vi "4_oop.vi"() -> ()   [LabVIEW 2024]
uses:
  <vilib>/Python/Open Venv Python Session.vi
panel:
  in  "Place":string(combo)="Baden, CH"
  out "Temperature [°C]":dbl
  in  "stop":bool
  # "The Independent Graphical Developer Conference\n11-13 September 2024\nStuttgart, Germany"
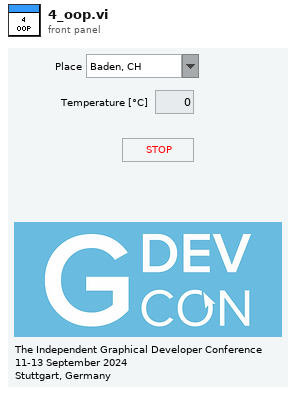
[diagram p1: front panel]
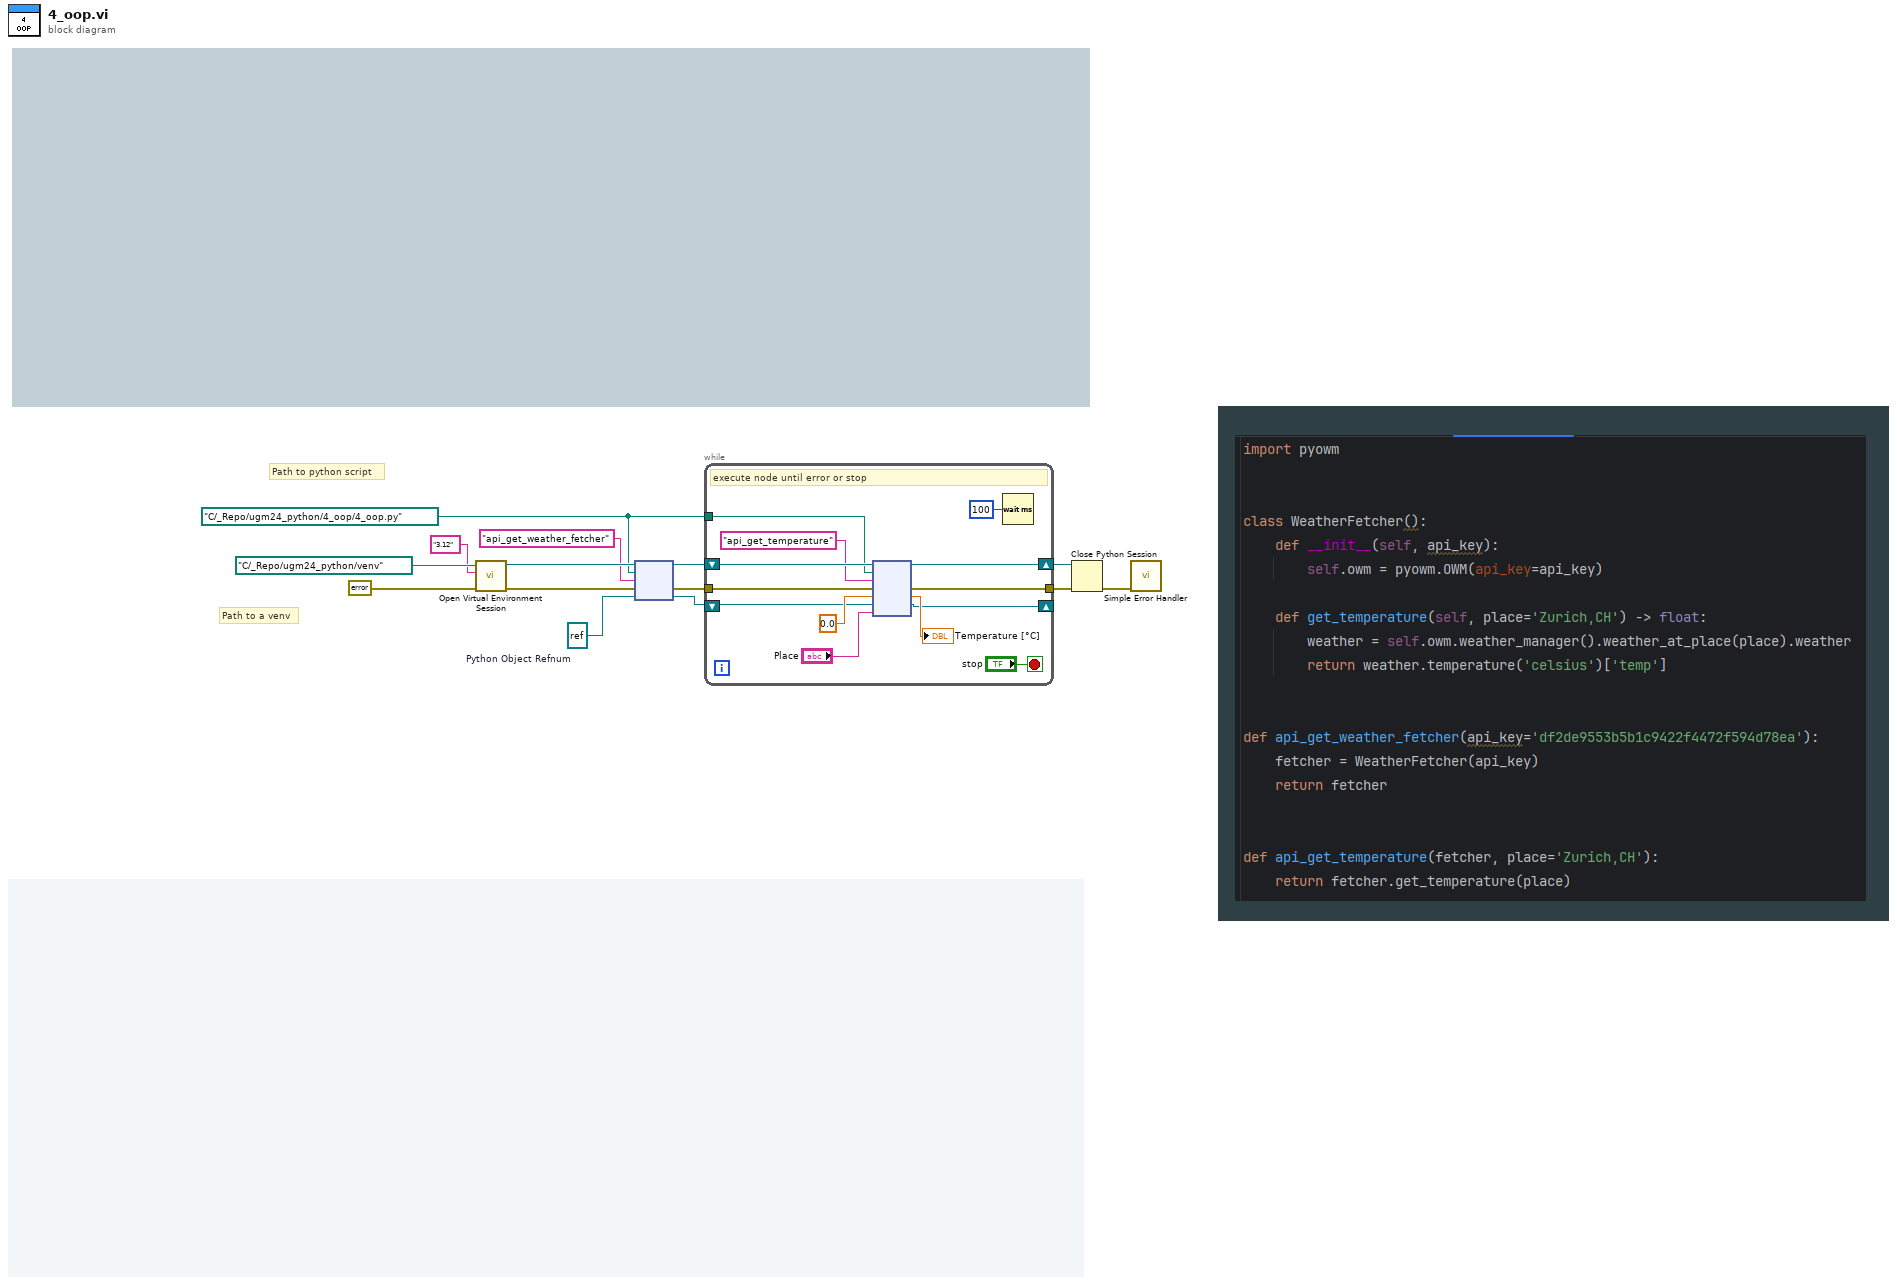
[diagram p0: block diagram]
diagram:
  w6 = refnum<k38> refnum  # Python Object Refnum
  w4 = path "C:/_Repo/ugm24_python/4_oop/4_oop.py" ("Path")
  # "Path to a venv"
  # "Path to python script"
  n1 = call-poly <vilib>:"Open Virtual Environment Session.vi"("error in (no error)"=errorcluster {"status"=FALSE, "code"=0, "source"=""}, "Python version"="3.12", "Env path"=path "C:/_Repo/ugm24_python/venv") -> ("error out"=w8:errorcluster, "session out"=w7:refnum<k35>)  [unwired: 7 in]
  n2 = node(w7, w4, "api_get_weather_fetcher" ("function name"), w8, w6) -> (w2:refnum<k35>, w3:errorcluster, w1:refnum<k38>)  [unwired: 2 out]
  n3 = while {
    tunnel: w3 -> [w27]
    tunnel: w4 -> [w25]
    tunnel: [w23] -> w14
    shift-right: [w22] -> w13
    shift-left: w2 -> [w26]
    shift-right: [w15] -> _
    shift-left: w1 -> [w17]
    stop <- "stop" stop-if-true
    # "execute node until error or stop"
    n4 = node(w26, w25, "api_get_temperature" ("function name"), w27, 0.0 ("Temperature"), w17, "Place") -> (w22:refnum<k35>, w23:errorcluster, →"Temperature [°C]":dbl, w15:refnum<k38>)  [unwired: 1 in, 2 out]
    n5 = Wait (ms)(milliseconds to wait=u32 100) -> ()  [unwired: 1 out]
  }
  n6 = Close Python Session(session in=w13, error in=w14) -> (11:w12:errorcluster)
  n7 = call <vilib>:"Simple Error Handler.vi"("error in (no error)"=w12) -> ()  [unwired: 4 in, 5 out]
